vi "Prepare image colour.vi"(7 "Image control":refnum<vi>, 8 "error in":errorcluster, 11 "Left Image Palette":enum16{"Gray", "Red", "Green"}(ring)) -> (0 "error out":errorcluster, 1 "Color Palette":cluster{"Red":u8, "Green":u8, "Blue":u8}[](array[cluster]), 3 "Palette Type":u32)   [LabVIEW 2020]
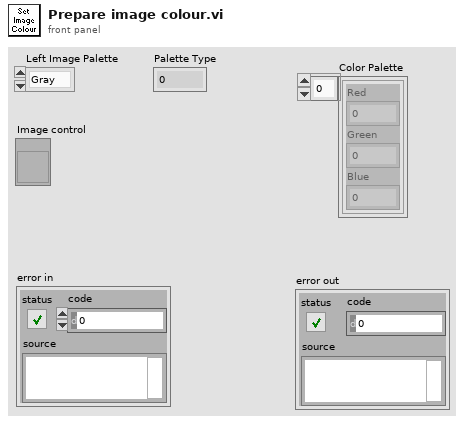
[diagram p1: front panel]
types:
  T1 = enum32{"Gray", "Binary", "Gradient", "Rainbow", "Temperature", "User Defined"}
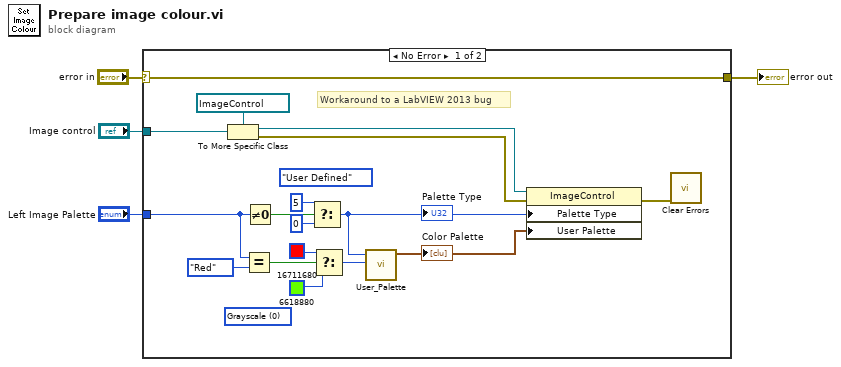
[diagram p0: block diagram]
diagram:
  n1 = case shown="No Error" "error in" {
    selector: "error in" -> [w5 w22]
    tunnel: "Left Image Palette" -> [w21 _]
    tunnel: "Image control" -> [w11 _]
    tunnel: [w5 w22] -> w1
    frame No Error {
      (unwired) u32 0 items=["Grayscale", "Binary", "Gradient", "Rainbow", "Temperature", "User Defined"] ("Palette:Palette Type")
      (unwired) T1."User Defined" ("Palette Number (gray)")
      # "Workaround to a LabVIEW 2013 bug"
      n2 = To More Specific Class(target class=refnum<vi> refnum ("Image"), reference=w11) -> (specific class reference=w10:refnum<vi>, error out=w7:errorcluster)  [unwired: 1 in]
      n3 = Equal?(x=w21, y=enum16{"Gray", "Red", "Green"}."Red") -> (x = y?=w18:bool)
      n4 = Not Equal To 0?(x=w21) -> (x != 0?=w13:bool)
      n5 = Select(t=u32 5, s=w13, f=u32 0) -> (s? t:f=w9:u32)
      "Palette Type" <- w9
      n6 = Select(t=u32 16711680 ("Color"), s=w18, f=u32 6618880 ("Color")) -> (s? t:f=w20:u32)
      n7 = call "User_Palette.vi"("Color"=w20, "Palette Number (gray)"=w9) -> ("Color Palette"=w8:cluster{"Red":u8, "Green":u8, "Blue":u8}[])  [unwired: 9 in]
      "Color Palette" <- w8
      n8 = property on="Property Node" class="ImageControl"(reference=w10, error in=w7, "Palette Type"=w9, "User Palette"=w8) -> (error out=w6:errorcluster)  [unwired: 1 out]
      n9 = call <vilib>:"Clear Errors.vi"("error in (no error)"=w6) -> ()  [unwired: 5 in, 2 out]
    }
    frame Error {
    }
  }
  "error out" <- w1
